vi "Measure timetrace.vi"(4 "error in":errorcluster, 5 "input main cluster":T1, 6 "Timetrace length (s)":i32, 7 "path":path) -> (0 "error out":errorcluster, 1 "output main cluster":T1, 3 "stoped?":bool)   [LabVIEW 2010]
uses:
  Main_cluster.ctl
  <vilib>/DAQmx/read.llb/DAQmx Read (Counter DBL 1Chan 1Samp).vi
  <vilib>/Utility/file.llb/Write To Spreadsheet File (DBL).vi
  <vilib>/daqmx/miscellaneous.llb/DAQmx Fill In Error Info.vi
panel:
  out "STOP":bool
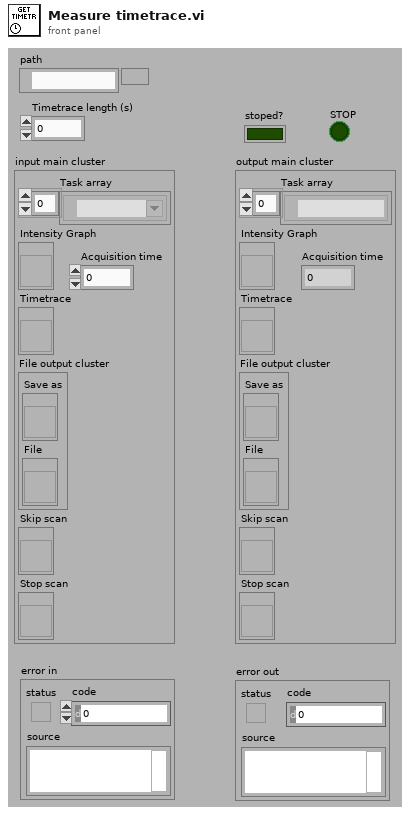
[diagram p1: front panel]
types:
  T1 = typedef "Main_cluster.ctl" = cluster{"Task array":refnum<k21>[], "Intensity Graph":refnum<vi>, "Timetrace":refnum<vi>, "File output cluster":cluster{"Save as":refnum<vi>, "File":refnum<vi>}, "Skip scan":refnum<vi>, "Stop scan":refnum<vi>, "Acquisition time":dbl}
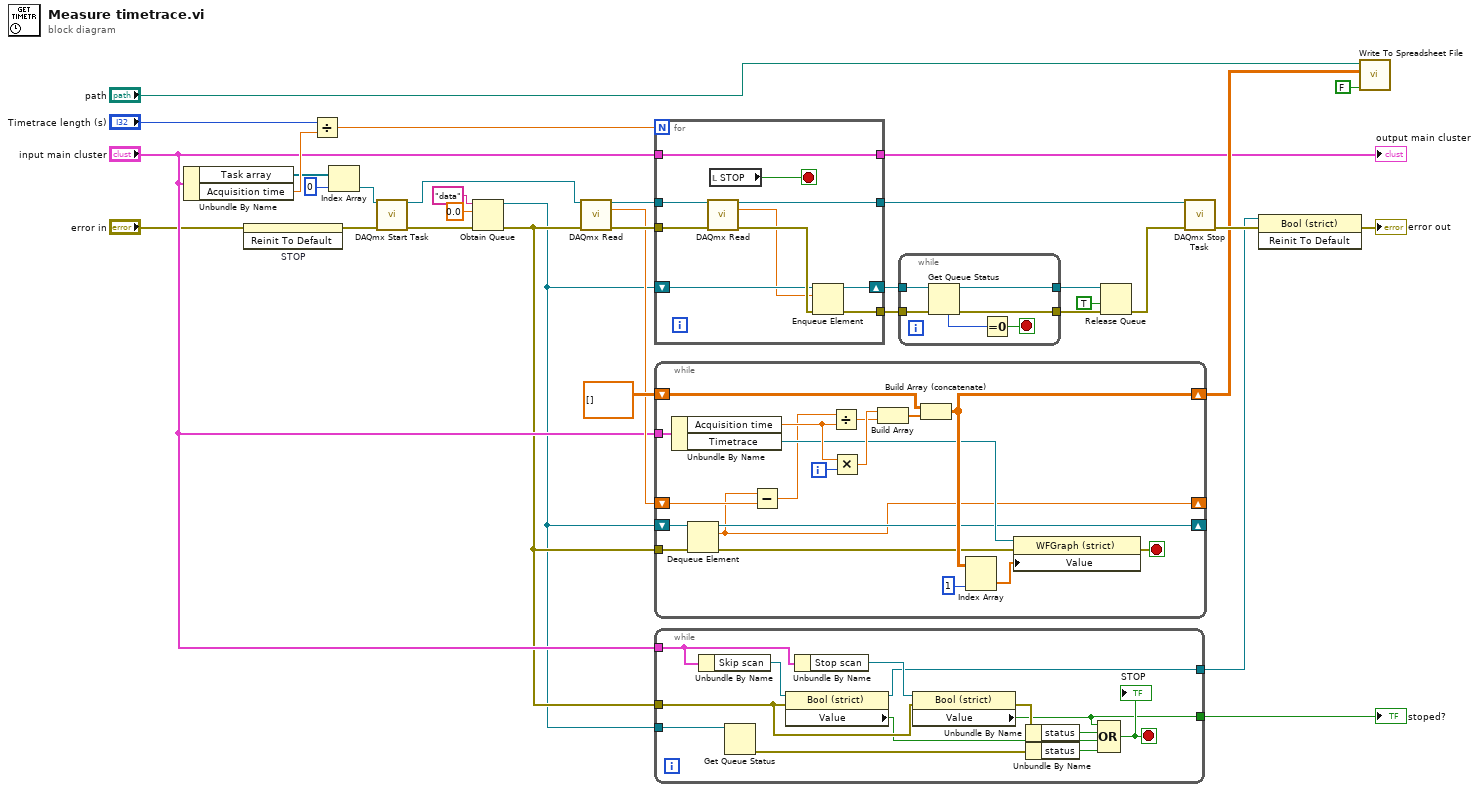
[diagram p0: block diagram]
diagram:
  n1 = Unbundle By Name("input main cluster") -> ("Task array"=w31:refnum<k21>[], "Acquisition time"=w34:dbl)
  n2 = invoke on="STOP" class="Bool (strict)" method="Reinit To Default"(error in="error in") -> (error out=w1:errorcluster)  [unwired: 2 in, 2 out]
  n3 = Divide(x="Timetrace length (s)", y=w34) -> (x/y=w24:dbl)
  n4 = Index Array(array=w31, index=0) -> (element=w33:refnum<k21>)
  n5 = call <vilib>:"DAQmx Start Task.vi"("task/channels in"=w33, "error in"=w1) -> ("task out"=w26:refnum<k21>, "error out"=w19:errorcluster)  [unwired: 12 out]
  n6 = Obtain Queue(name (unnamed)="data", element data type=0.0 ("data"), error in (no error)=w19) -> (queue out=w7:refnum<queue>, error out=w11:errorcluster)  [unwired: 2 in, 1 out]
  n7 = call-poly <vilib>:"DAQmx Read.vi"("task/channels in"=w26, "error in"=w11) -> ("task out"=w27:refnum<k21>, "data"=w17:dbl, "error out"=w23:errorcluster)  [unwired: 11 in]
  n8 = for {
    N: w24 -> [_]
    tunnel: w23 -> [w44]
    tunnel: w27 -> [w43]
    tunnel: "input main cluster" -> [w35]
    shift-right: [w39] -> w16
    shift-left: w7 -> [w41]
    tunnel: [w38] -> w4
    tunnel: [w37] -> w10
    tunnel: [w35] -> w6
    stop <- w36 stop-if-true
    n9 = call-poly <vilib>:"DAQmx Read.vi"("task/channels in"=w43, "error in"=w44) -> ("task out"=w37:refnum<k21>, "data"=w40:dbl, "error out"=w42:errorcluster)  [unwired: 11 out]
    n10 = local read "STOP"() -> (w36:bool)
    n11 = Enqueue Element(queue=w41, element=w40, error in (no error)=w42) -> (queue out=w39:refnum<queue>, error out=w38:errorcluster)  [unwired: 1 in, 1 out]
  }
  "output main cluster" <- w6
  n12 = while {
    shift-right: [w48] -> _
    shift-left: w17 -> [w63]
    shift-right: [w58] -> w14
    shift-left: dbl[][] [] -> [w60]
    tunnel: "input main cluster" -> [w53]
    tunnel: w11 -> [w51]
    shift-right: [w49] -> _
    shift-left: w7 -> [w50]
    i -> [w62]
    stop <- w47 stop-if-true
    n13 = Unbundle By Name(w53) -> ("Acquisition time"=w55:dbl, "Timetrace"=w54:refnum<vi>)
    n14 = Dequeue Element(queue=w50, error in (no error)=w51) -> (queue out=w49:refnum<queue>, element=w48:dbl, error out=w52:errorcluster)  [unwired: 1 in, 1 out]
    n15 = Subtract(x=w48, y=w63) -> (x-y=w46:dbl)
    n16 = Divide(x=w46, y=w55) -> (x/y=w45:dbl)
    n17 = Multiply(x=w55, y=w62) -> (x*y=w61:dbl)
    n18 = Build Array(w61, w45) -> (w59:dbl[])
    n19 = Build Array (concatenate)(w60, w59) -> (w58:dbl[][])
    n20 = Index Array(array=w58, index (col)=1 ("index (row)")) -> (element=w56:dbl[])  [unwired: 1 in]
    n21 = property on="Property Node" class="WFGraph (strict)"(reference=w54, error in=w52, "Value"=w56) -> (error out=w47:errorcluster)  [unwired: 1 out]
  }
  n22 = while {
    tunnel: "input main cluster" -> [w72]
    tunnel: w11 -> [w71]
    tunnel: [w68] -> w9
    tunnel: [w67] -> w8
    tunnel: w7 -> [w66]
    stop <- w69 stop-if-true
    n23 = Unbundle By Name(w72) -> ("Skip scan"=w74:refnum<vi>)
    n24 = Get Queue Status(queue=w66) -> (error out=w65:errorcluster)  [unwired: 2 in, 7 out]
    n25 = property class="Bool (strict)"(reference=w74, error in=w71) -> (reference out=w68:refnum<vi>, "Value"=w70:bool)  [unwired: 1 out]
    n26 = Unbundle By Name(w72) -> ("Stop scan"=w73:refnum<vi>)
    n27 = property class="Bool (strict)"(reference=w73, error in=w71) -> (error out=w75:errorcluster, "Value"=w67:bool)  [unwired: 1 out]
    n28 = Unbundle By Name(w75) -> ("status"=w76:bool)
    n29 = Unbundle By Name(w65) -> ("status"=w64:bool)
    n30 = Compound Arithmetic op=OR(w67, w76, w70, w64) -> (w69:bool)
    "STOP" <- w69
  }
  "stoped?" <- w8
  n31 = while {
    tunnel: w16 -> [w82]
    tunnel: [w81] -> w5
    tunnel: w4 -> [w80]
    tunnel: [w79] -> w3
    stop <- w77 stop-if-true
    n32 = Get Queue Status(queue=w82, error in (no error)=w80) -> (queue out=w81:refnum<queue>, error out=w79:errorcluster, # elements in queue=w78:i32)  [unwired: 1 in, 5 out]
    n33 = Equal To 0?(x=w78) -> (x = 0?=w77:bool)
  }
  n34 = Release Queue(queue=w5, force destroy? (F)=TRUE, error in (no error)=w3) -> (error out=w15:errorcluster)  [unwired: 2 out]
  n35 = call <vilib>:"DAQmx Stop Task.vi"("task/channels in"=w10, "error in"=w15) -> ("error out"=w29:errorcluster)  [unwired: 13 out]
  n36 = invoke on="Invoke Node" class="Bool (strict)" method="Reinit To Default"(reference=w9, error in=w29) -> (error out=→"error out":errorcluster)  [unwired: 1 in, 2 out]
  n37 = call-poly <vilib>:"Write To Spreadsheet File.vi"("append to file? (new file:F)"=FALSE, "2D data"=w14, "file path (dialog if empty)"="path") -> ()  [unwired: 5 in, 1 out]
